vi "DMM.vi"(8 "error in":errorcluster, 9 "Setting":T1={"Resolution (Digits)"=5.5, "Current Source (Amps)"=0.001, "Range"=2.0, "Measurement Type"=enum."DC Volts"} {"Resolution (Digits)" items=["3 1/2"=3.5, "4 1/2"=4.5, "5 1/2"=5.5, "6 1/2"=6.5, "7 1/2"=7.5]; "Current Source (Amps)" items=["1uA"=1e-06, "10uA"=1e-05, "100uA"=0.0001, "1mA"=0.001]}, 10 "DMM Ref":string="NI_DMM_4072", 11 "DMM":refnum<class "MIO.lvclass">) -> (0 "error out":errorcluster={"status"=TRUE, "code"=7, "source"="Get LV Class Default Value.vi<APPEND>\n\n<b>Complete call chain:</b>\r\n     Get LV Class Default Value.vi\r\n     MAL.lvlib:DMM.vi\r\n\r\n<b>LabVIEW attempted to load the class at this path:</b>\r\nC:\\GitHub\\OOP Template\\HAL\\Concrete\\NI DMM4072.lvclass\\NI DMM4072.lvclass.lvclass"}, 2 "Measurements":dbl, 3 "DMM":refnum<class "MIO.lvclass">)   [LabVIEW 2019, in "Measuremtn Abstraction.lvlib"]
uses:
  Measuremtn Abstraction.lvlib
  Hardware Abstraction/Harware Abstraction/MultiIO/MIO.lvclass
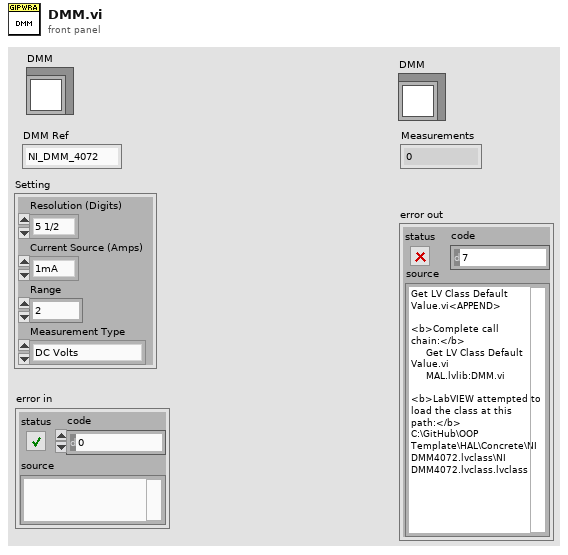
[diagram p1: front panel]
types:
  T1 = cluster{"Resolution (Digits)":dbl, "Current Source (Amps)":dbl, "Range":dbl, "Measurement Type":enum16{"DC Volts", "AC Volts", "DC Current", "AC Current", "2-wire Resistance", "4-wire Resistance", "Diode", "Frequency", "Period", "AC Volts DC Coupled", "Capacitance", "Inductance", "Temperature"}}
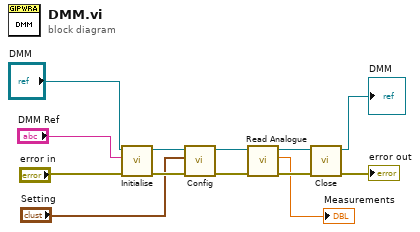
[diagram p0: block diagram]
diagram:
  n1 = call-dynamic "Initialise.vi"("error in (no error)"="error in", "Instrument Ref"="DMM Ref", "Instrument in"="DMM") -> ("error out"=w13:errorcluster, "Instrument out"=w10:refnum<class "MIO.lvclass">)  [unwired: 7 in]
  n2 = call-dynamic "Config.vi"("error in (no error)"=w13, "Setting"="Setting", "DMM in"=w10) -> ("error out"=w12:errorcluster, "DMM out"=w9:refnum<class "MIO.lvclass">)  [unwired: 7 in]
  n3 = call-dynamic "Read Analogue.vi"("error in (no error)"=w12, "DMM in"=w9) -> ("error out"=w11:errorcluster, "Measurement"=→"Measurements":dbl, "DMM out"=w8:refnum<class "MIO.lvclass">)  [unwired: 7 in]
  n4 = call-dynamic "Close.vi"("error in (no error)"=w11, "Instrument in"=w8) -> ("error out"=→"error out":errorcluster, "Instrument out"=→"DMM":refnum<class "MIO.lvclass">)  [unwired: 8 in]
